vi "U01_4_AutomaticConnection.vi"() -> ()   [LabVIEW 2015]
panel:
  in  "Tab Control":enum32{"Page 1", "Page 2"}(tab)
  in  "Port":u16=80
  in  "IP":string
  in  "BtnExit":bool
  out "error out":errorcluster
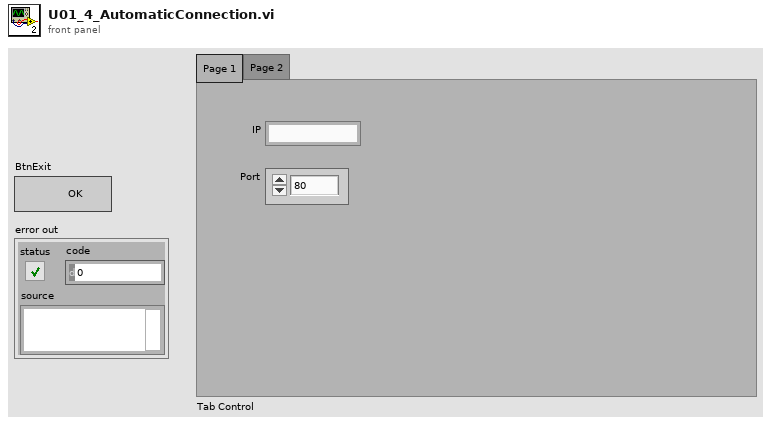
[diagram p1: front panel]
types:
  T1 = cluster{"Message":string, "TCPCL":cluster{"connection ID":refnum<k5>, "ID":u16}}
  T2 = cluster{"connection ID":refnum<k5>, "service name":string, "port":u16}
  T3 = cluster{"Message":string, "ID":i32, "TCPCL":cluster{"connection ID":refnum<k5>, "service name":string, "port":u16}}
  T4 = cluster{string, "TCPCL":cluster{"connection ID":refnum<k5>, "port":u16}}
  T5 = cluster{string, "TCPCL":cluster{"connection ID":refnum<k5>, "ID":u16}}
  T6 = cluster{"connection ID":refnum<k5>, "Value":string, "Value":u16}
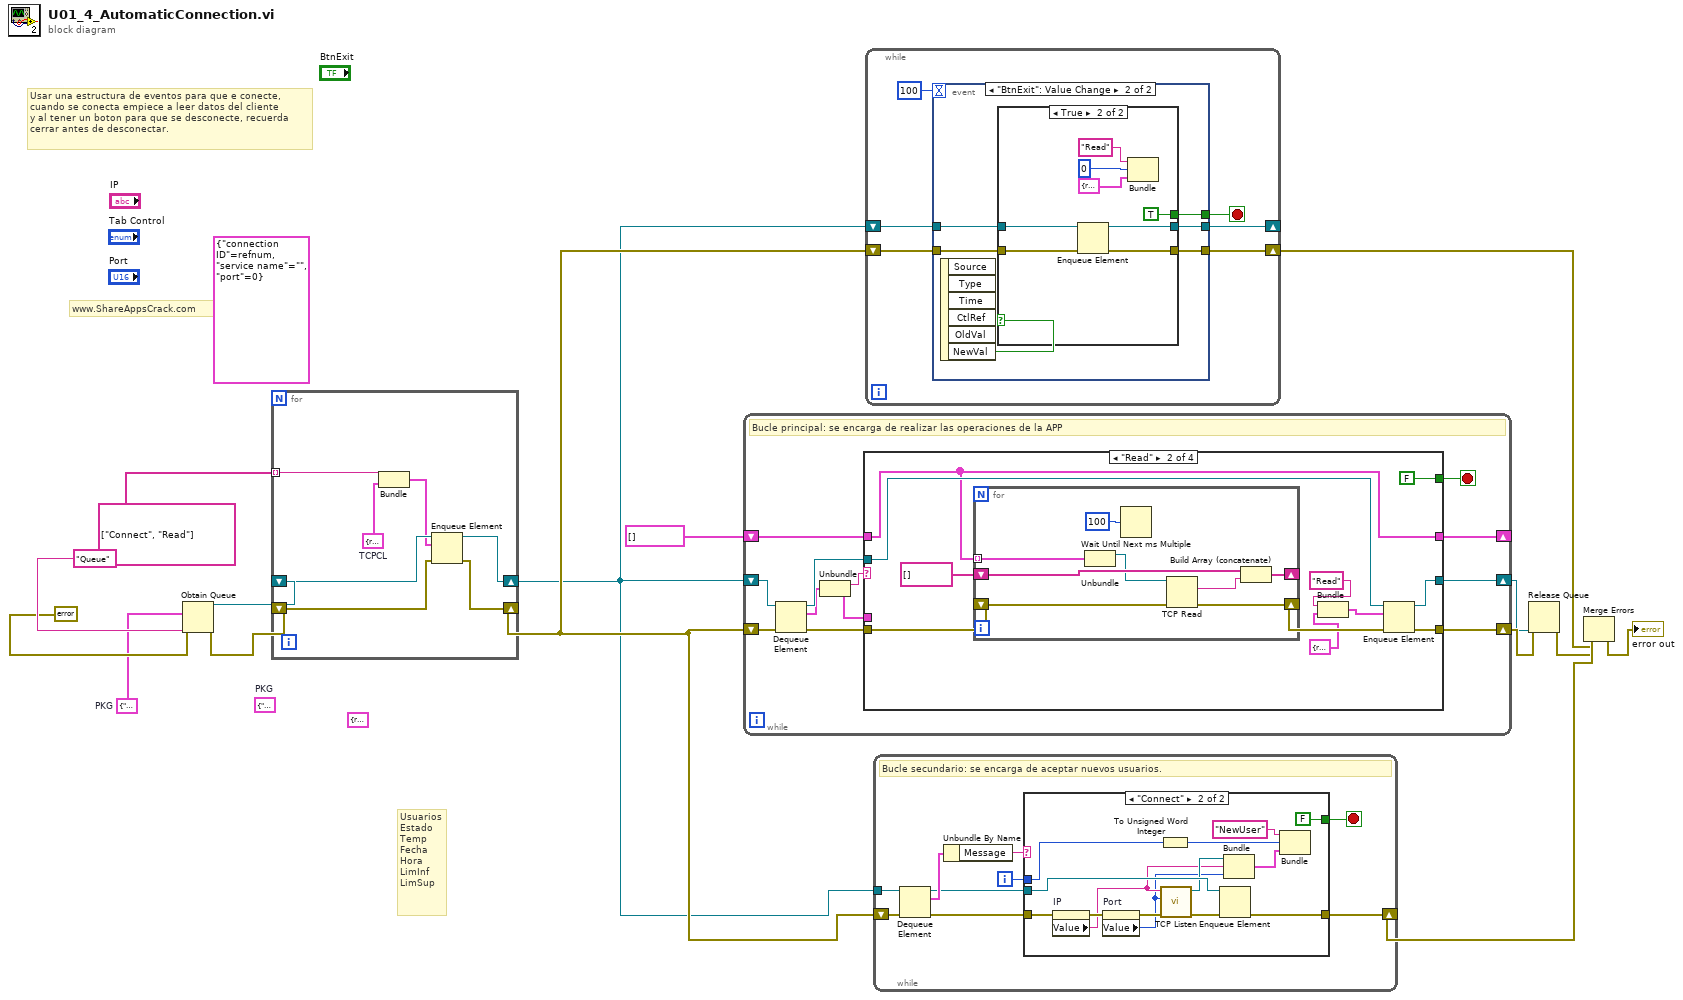
[diagram p0: block diagram]
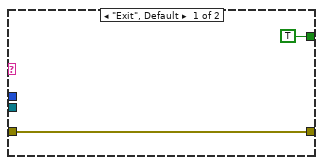
[diagram p2: hidden frame]
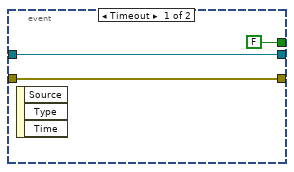
[diagram p3: hidden frame]
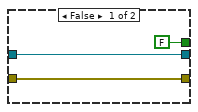
[diagram p4: hidden frame]
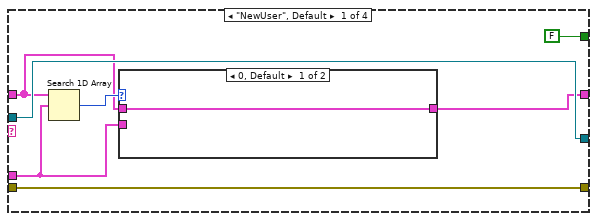
[diagram p5: hidden frame]
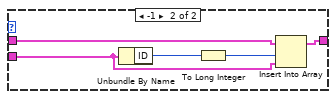
[diagram p6: hidden frame]
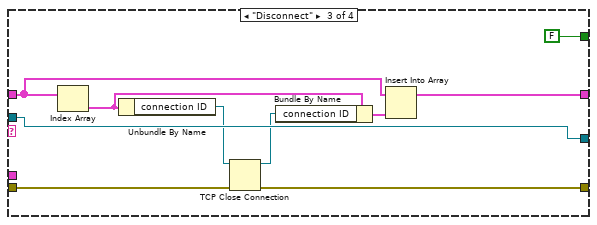
[diagram p7: hidden frame]
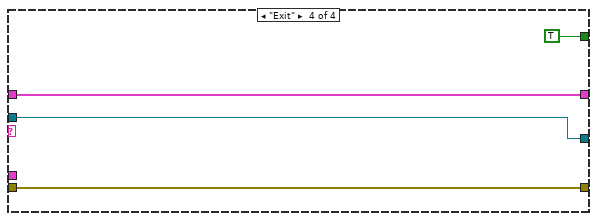
[diagram p8: hidden frame]
diagram:
  w1 = T1 {"Message"="", "TCPCL"={"connection ID"=refnum, "ID"=0}}  # PKG
  (unwired) cluster{"connection ID":refnum<k5>, "ID":u16} {"connection ID"=refnum, "ID"=0} ("TCPCL")
  (unwired) T2 {"connection ID"=refnum, "service name"="", "port"=0} ("TCPCL")
  (unwired) T3 {"Message"="", "ID"=0, "TCPCL"={"connection ID"=refnum, "service name"="", "port"=0}}  # PKG
  # "Usuarios\nEstado\nTemp\nFecha\nHora\nLimInf\nLimSup"
  # "Usar una estructura de eventos para que e conecte,\ncuando se conecta empiece a leer datos del cliente\ny al tener un boton para que se desconecte, recuerda \ncerrar antes de desconectar."
  # "www.ShareAppsCrack.com"
  n1 = Obtain Queue(name (unnamed)="Queue", element data type=w1, error in (no error)=errorcluster {"status"=FALSE, "code"=0, "source"=""}) -> (queue out=w13:refnum<queue>, error out=w12:errorcluster)  [unwired: 2 in, 1 out]
  n2 = for {
    shift-right: [w18] -> w8
    shift-left: w13 -> [w21]
    shift-right: [w19] -> w9
    shift-left: w12 -> [w20]
    tunnel: string[] ["Connect", "Read"] -> [w22] mode=indexing
    w17 = cluster{"connection ID":refnum<k5>, "port":u16} {"connection ID"=refnum, "port"=0}  # TCPCL
    n3 = Bundle(w22, "TCPCL"=w17) -> (w16:T4)  [unwired: 1 in]
    n4 = Enqueue Element(queue=w21, element=w16, error in (no error)=w20) -> (queue out=w18:refnum<queue>, error out=w19:errorcluster)  [unwired: 1 in, 1 out]
  }
  n5 = while {
    shift-right: [w33] -> w6
    shift-left: w9 -> [w29]
    shift-right: [w34] -> w4
    shift-left: w8 -> [w31]
    shift-right: [w25] -> _
    shift-left: cluster{"connection ID":refnum<k5>, "ID":u16}[] [] -> [w24]
    stop <- w32 stop-if-true
    # "Bucle principal: se encarga de realizar las operaciones de la APP"
    n6 = Dequeue Element(queue=w31, error in (no error)=w29) -> (queue out=w30:refnum<queue>, element=w27:T1, error out=w28:errorcluster)  [unwired: 1 in, 1 out]
    n7 = Unbundle(w27) -> ("Message"=w26:string, "TCPCL"=w23:cluster{"connection ID":refnum<k5>, "ID":u16})
    n8 = case shown="\"Read\"" w26 {
      tunnel: w28 -> [w39 w58 w75 w79]
      tunnel: w30 -> [w40 w57 w76 w78]
      tunnel: [w40 w56 w76 w78] -> w34
      tunnel: [w39 w54 w74 w79] -> w33
      tunnel: [FALSE ("status") FALSE FALSE TRUE] -> w32
      tunnel: [w35 w51 w67 w77] -> w25
      tunnel: w24 -> [w36 w51 w69 w77]
      tunnel: w23 -> [w38 _ _ _]
      frame "NewUser", Default {
        n9 = Search 1D Array(1D array=w36, element=w38) -> (index of element=w37:i32)  [unwired: 1 in]
        n10 = case shown="0, Default" w37 {
          tunnel: w36 -> [w42 w47]
          tunnel: w38 -> [_ w46]
          tunnel: [w42 w43] -> w35
          frame 0, Default {
          }
          frame -1 {
            n11 = Unbundle By Name(w46) -> ("ID"=w45:u16)
            n12 = To Long Integer(number=w45) -> (32bit integer=w44:i32)
            n13 = Insert Into Array(array=w47, index=w44, new element=w46) -> (w43:cluster{"connection ID":refnum<k5>, "ID":u16}[])
          }
        }
      }
      frame "Read" {
        n14 = for {
          shift-right: [w65] -> w55
          shift-left: w58 -> [w66]
          tunnel: w51 -> [w61] mode=indexing
          shift-right: [w63] -> _
          shift-left: string[] [] -> [w64]
          n15 = Unbundle(w61) -> ("connection ID"=w60:refnum<k5>)  [unwired: 1 out]
          n16 = Wait Until Next ms Multiple(millisecond multiple=u32 100) -> ()  [unwired: 1 out]
          n17 = TCP Read(connection ID=w60, error in (no error)=w66) -> (data out=w62:string, error out=w65:errorcluster)  [unwired: 3 in, 1 out]
          n18 = Build Array (concatenate)(w64, w62) -> (w63:string[])
        }
        n19 = Bundle("Read", "TCPCL"=cluster{"connection ID":refnum<k5>, "ID":u16} {"connection ID"=refnum, "ID"=0}) -> (w48:T5)  [unwired: 1 in]
        n20 = Enqueue Element(queue=w57, element=w48, error in (no error)=w55) -> (queue out=w56:refnum<queue>, error out=w54:errorcluster)  [unwired: 1 in, 1 out]
      }
      frame "Disconnect" {
        n21 = Index Array(array=w69) -> (element=w70:cluster{"connection ID":refnum<k5>, "ID":u16})  [unwired: 1 in]
        n22 = Unbundle By Name(w70) -> ("connection ID"=w71:refnum<k5>)
        n23 = TCP Close Connection(connection ID=w71, error in (no error)=w75) -> (connection ID out=w73:refnum<k5>, error out=w74:errorcluster)  [unwired: 1 in]
        n24 = Bundle By Name(cluster=w70, "connection ID"=w73) -> (w68:cluster{"connection ID":refnum<k5>, "ID":u16})
        n25 = Insert Into Array(array=w69, new element=w68) -> (w67:cluster{"connection ID":refnum<k5>, "ID":u16}[])  [unwired: 1 in]
      }
      frame "Exit" {
      }
    }
  }
  n26 = while {
    shift-right: [w82] -> _
    shift-left: w8 -> [w85]
    shift-right: [w81] -> w3
    shift-left: w9 -> [w84]
    stop <- w83 stop-if-true
    n27 = event shown="[1] \"BtnExit\": Value Change" {
      selector: _ -> [_ _]
      dyn-events: _ -> [_ _]
      timeout: 100 -> [_ _]
      tunnel: w85 -> [w88 w94]
      tunnel: w84 -> [w87 w93]
      tunnel: [FALSE w92] -> w83
      tunnel: [w88 w91] -> w82
      tunnel: [w87 w90] -> w81
      event Timeout {
        n28 = event-data() -> ()  [unwired: 1 in, 3 out]
      }
      event "BtnExit": Value Change {
        n29 = event-data() -> ("NewVal"=w95:bool)  [unwired: 1 in, 5 out]
        n30 = case shown="True" w95 {
          tunnel: w94 -> [w96 w103]
          tunnel: w93 -> [w97 w102]
          tunnel: [FALSE TRUE] -> w92
          tunnel: [w96 w100] -> w91
          tunnel: [w97 w99] -> w90
          frame False {
          }
          frame True {
            n31 = Enqueue Element(queue=w103, error in (no error)=w102) -> (queue out=w100:refnum<queue>, error out=w99:errorcluster)  [unwired: 2 in, 1 out]
            n32 = Bundle("Read", 0, "TCPCL"=T2 {"connection ID"=refnum, "service name"="127.0.0.1", "port"=80}) -> ()  [unwired: 1 in, 1 out]
          }
        }
      }
    }
  }
  n33 = while {
    tunnel: w8 -> [w114]
    shift-right: [w110] -> w7
    shift-left: w9 -> [w115]
    i -> [w107]
    stop <- w109 stop-if-true
    # "Bucle secundario: se encarga de aceptar nuevos usuarios."
    n34 = Dequeue Element(queue=w114, error in (no error)=w115) -> (queue out=w108:refnum<queue>, element=w113:T1, error out=w111:errorcluster)  [unwired: 1 in, 1 out]
    n35 = Unbundle By Name(w113) -> ("Message"=w112:string)
    n36 = case shown="\"Connect\"" w112 {
      tunnel: [w117 w125] -> w110
      tunnel: w111 -> [w117 w131]
      tunnel: [TRUE FALSE] -> w109
      tunnel: w108 -> [_ w127]
      tunnel: w107 -> [_ w119]
      frame "Exit", Default {
      }
      frame "Connect" {
        n37 = property on="IP" class="Str"(error in=w131) -> (error out=w130:errorcluster, "Value"=w121:string)  [unwired: 1 in, 1 out]
        n38 = property on="Port" class="DigNum (strict)"(error in=w130) -> (error out=w129:errorcluster, "Value"=w120:u16)  [unwired: 1 in, 1 out]
        n39 = To Unsigned Word Integer(number=w119) -> (unsigned 16bit integer=w118:u16)
        n40 = call <vilib>:"TCP Listen.vi"("error in (no error)"=w129, "port"=w120, "service name"=w121) -> ("error out"=w126:errorcluster, "connection ID"=w122:refnum<k5>)  [unwired: 4 in, 3 out]
        n41 = Enqueue Element(queue=w127, error in (no error)=w126) -> (error out=w125:errorcluster)  [unwired: 2 in, 2 out]
        n42 = Bundle("connection ID"=w122, "Value"=w121, "Value"=w120) -> (w123:T6)  [unwired: 1 in]
        n43 = Bundle("NewUser", w118, w123) -> ()  [unwired: 1 in, 1 out]
      }
    }
  }
  n44 = Release Queue(queue=w4, error in (no error)=w6) -> (error out=w5:errorcluster)  [unwired: 1 in, 2 out]
  n45 = Merge Errors(w3, w5, w7) -> (→"error out":errorcluster)
